vi "AR-msg-vars-FGV.vi"(7 "Action":enum16{"Init", "WR", "RD"}(ring), 8 "error in":errorcluster, 11 "msg-var in":T1) -> (0 "error out":errorcluster, 3 "msg-var":T1)   [LabVIEW 2021]
uses:
  Controls/AR-msg-variables.ctl
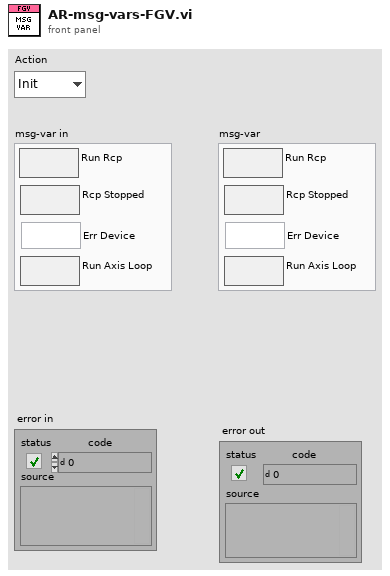
[diagram p1: front panel]
types:
  T1 = typedef "AR-msg-variables.ctl" = cluster{"Run Rcp":bool, "Rcp Stopped":bool, "Err Device":string, "Run Axis Loop":bool}
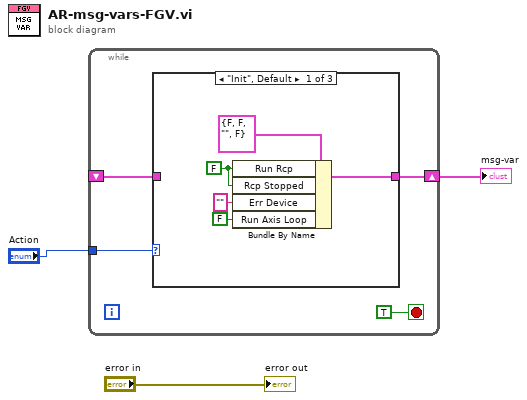
[diagram p0: block diagram]
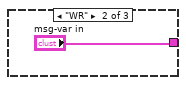
[diagram p2: hidden frame]
diagram:
  n1 = while {
    tunnel: "Action" -> [w6]
    shift-right: [w5] -> w2
    shift-left: _ -> [w4]
    stop <- TRUE stop-if-true
    n2 = case shown="\"Init\", Default" w6 {
      tunnel: [w11 "msg-var in" w14] -> w5
      tunnel: w4 -> [_ _ w14]
      frame "Init", Default {
        w10 = FALSE ("Run Rcp")
        n3 = Bundle By Name(cluster=T1 {"Run Rcp"=FALSE, "Rcp Stopped"=FALSE, "Err Device"="", "Run Axis Loop"=FALSE} ("msg-var"), "Run Rcp"=w10, "Rcp Stopped"=w10, "Err Device"="", "Run Axis Loop"=FALSE ("Settings")) -> (w11:T1)
      }
      frame "WR" {
      }
      frame "RD" {
      }
    }
  }
  "msg-var" <- w2
  "error out" <- "error in"
